vi "tm_opencamera.vi"(7 "Force Open":bool, 8 "error in (no error)":errorcluster, 11 "Camera Index":u32) -> (0 "error out":errorcluster, 3 "Handle out":u32)   [LabVIEW 2015]
uses:
  tmcamcon.dll
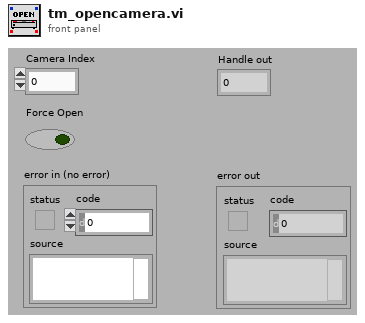
[diagram p1: front panel]
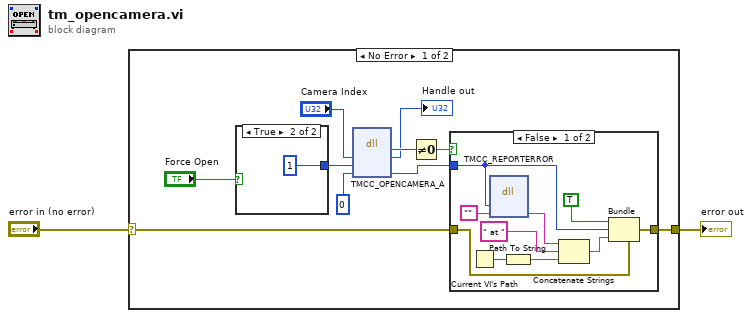
[diagram p0: block diagram]
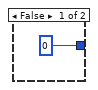
[diagram p2: hidden frame]
diagram:
  n1 = case shown="No Error" "error in (no error)" {
    selector: "error in (no error)" -> [w6 w26]
    tunnel: [w5 w26] -> w1
    frame No Error {
      n2 = case shown="True" "Force Open" {
        tunnel: [0 1] -> w3
        frame False {
        }
        frame True {
        }
      }
      n3 = dll-call lib="tmcamcon.dll" fn="TMCC_OPENCAMERA_A"("i"="Camera Index", "force"=w3, "Erval"=0) -> ("return type"=w12:u32, "i"=→"Handle out":u32, "Erval"=w8:i32)  [unwired: 4 in, 2 out]
      n4 = Not Equal To 0?(x=w12) -> (x != 0?=w7:bool)
      n5 = case shown="False" w7 {
        tunnel: w6 -> [w24 w25]
        tunnel: [w23 w25] -> w5
        tunnel: w8 -> [w17 _]
        frame False {
          n6 = Current VI's Path() -> (path=w22:path)
          n7 = dll-call lib="tmcamcon.dll" fn="TMCC_REPORTERROR"("error"=w17, "buf"="") -> ("buf"=w16:string)  [unwired: 5 in, 2 out]
          n8 = Path To String(path=w22) -> (string=w18:string)
          n9 = Concatenate Strings(w16, " at ", w18) -> (w21:string)
          n10 = Bundle(cluster=w24, "status"=TRUE, "code"=w17, "source"=w21) -> (w23:errorcluster)
        }
        frame True {
        }
      }
    }
    frame Error {
    }
  }
  "error out" <- w1
